vi "Write Task.vi"(8 "error in (no error)":errorcluster, 10 "Task":refnum<k21>, 11 "Thermometer DAQmx Config in":refnum<class "Thermometer DAQmx Config.lvclass">) -> (0 "error out":errorcluster, 3 "Thermometer DAQmx Config out":refnum<class "Thermometer DAQmx Config.lvclass">)   [LabVIEW 2023, in "Thermometer.lvlib" / "Thermometer DAQmx.lvlib" / "Thermometer DAQmx Config.lvclass"]
uses:
  Thermometer DAQmx Config.lvclass
  Thermometer DAQmx Config.lvclass/Thermometer DAQmx Config.ctl
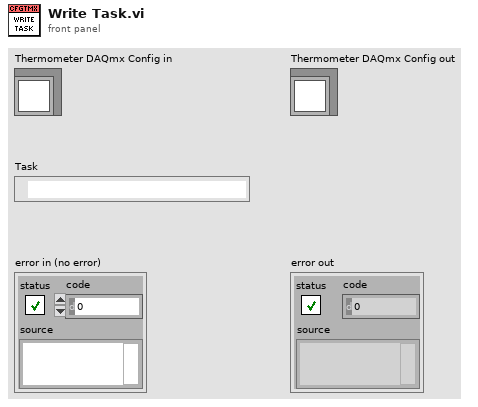
[diagram p1: front panel]
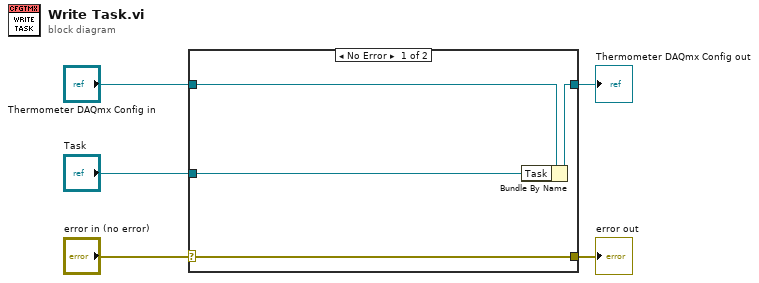
[diagram p0: block diagram]
diagram:
  n1 = case shown="No Error" "error in (no error)" {
    selector: "error in (no error)" -> [w9 w10]
    tunnel: [w9 w10] -> w4
    tunnel: [w7 w11] -> w2
    tunnel: "Thermometer DAQmx Config in" -> [w8 w11]
    tunnel: "Task" -> [w6 _]
    frame No Error {
      n2 = Bundle By Name(cluster=w8, "Task"=w6) -> (w7:refnum<class "Thermometer DAQmx Config.lvclass">)
    }
    frame Error {
    }
  }
  "error out" <- w4
  "Thermometer DAQmx Config out" <- w2
